vi "Autonomous Independent.vi"   [LabVIEW 2020]
doc: "This VI is called when autonomous begins, and will automatically be terminated when autonomous ends. You can carry out timed or sensor driven robot movement independently without needing to return to the caller."
uses:
  <vilib>/Rock Robotics/WPI/Solenoid/WPI_SolenoidValue.ctl
  <vilib>/Rock Robotics/WPI/Utilities/WPI_GetSetVariantRefNum.vi
  <vilib>/Rock Robotics/Network Tables/NT Read String.vi
  <vilib>/Rock Robotics/Network Tables/NT Write Numeric Array.vi
  Robot Global Data.vi
  <vilib>/Rock Robotics/Network Tables/NT Read Boolean.vi
  <vilib>/Rock Robotics/Network Tables/NT Read Number.vi
  Dawgma Programming Library/Utilities/armSetpoints.vi
  <vilib>/Rock Robotics/WPI/Solenoid/WPI_SolenoidSetEnum.vi
panel:
  # "Math for the\nfirst operation"
types:
  T1 = typedef "WPI_JoystickDevRef.ctl" = cluster{"Device":T2}
  T2 = typedef "WPI_JoystickDeviceEnum.ctl" = enum16{"USB 0", "USB 1", "USB 2", "USB 3", "USB 4", "USB 5"}
  T3 = typedef "WPI_SolenoidValue.ctl" = enum16{"Off", "On", "Forward", "Reverse"}
  T4 = typedef "Trajectory_Library.lvlib/SWERVE_DRIVE_ODOMETRY.ctl" = cluster{"POSE":T5, "GyroOffset":T7, "PreviousAngle":T7, "PrevModulePositions":T8[], "NumModules":i32}
  T5 = typedef "Trajectory_Library.lvlib/POSE2D.ctl" = cluster{"TRANSLATION":T6, "ROTATION":T7}
  T6 = typedef "Trajectory_Library.lvlib/TRANSLATION2D.ctl" = cluster{"X":dbl, "Y":dbl}
  T7 = typedef "Trajectory_Library.lvlib/ROTATION2D.ctl" = cluster{"VALUE":dbl, "COS":dbl, "SIN":dbl}
  T8 = typedef "Trajectory_Library.lvlib/SWERVE_DRIVE_MODULE_POSITION.ctl" = cluster{"Distance":dbl, "Angle":T7, "P":bool}
  T9 = typedef "WPI_SolenoidDevRef.ctl" = cluster{"DevStatus":errorcluster, "Pneumatics Control Module":u8, "Forward Solenoid Channel":T10, "Reverse Solenoid Channel":T10}
  T10 = typedef "WPI_SolenoidChannel.ctl" = enum8{"Solenoid 0", "Solenoid 1", "Solenoid 2", "Solenoid 3", "Solenoid 4", "Solenoid 5", "Solenoid 6", "Solenoid 7", "Solenoid 8", "Solenoid 9", "Solenoid 10", "Solenoid 11", "Solenoid 12", "Solenoid 13", "Solenoid 14", "Solenoid 15", "Invalid"}
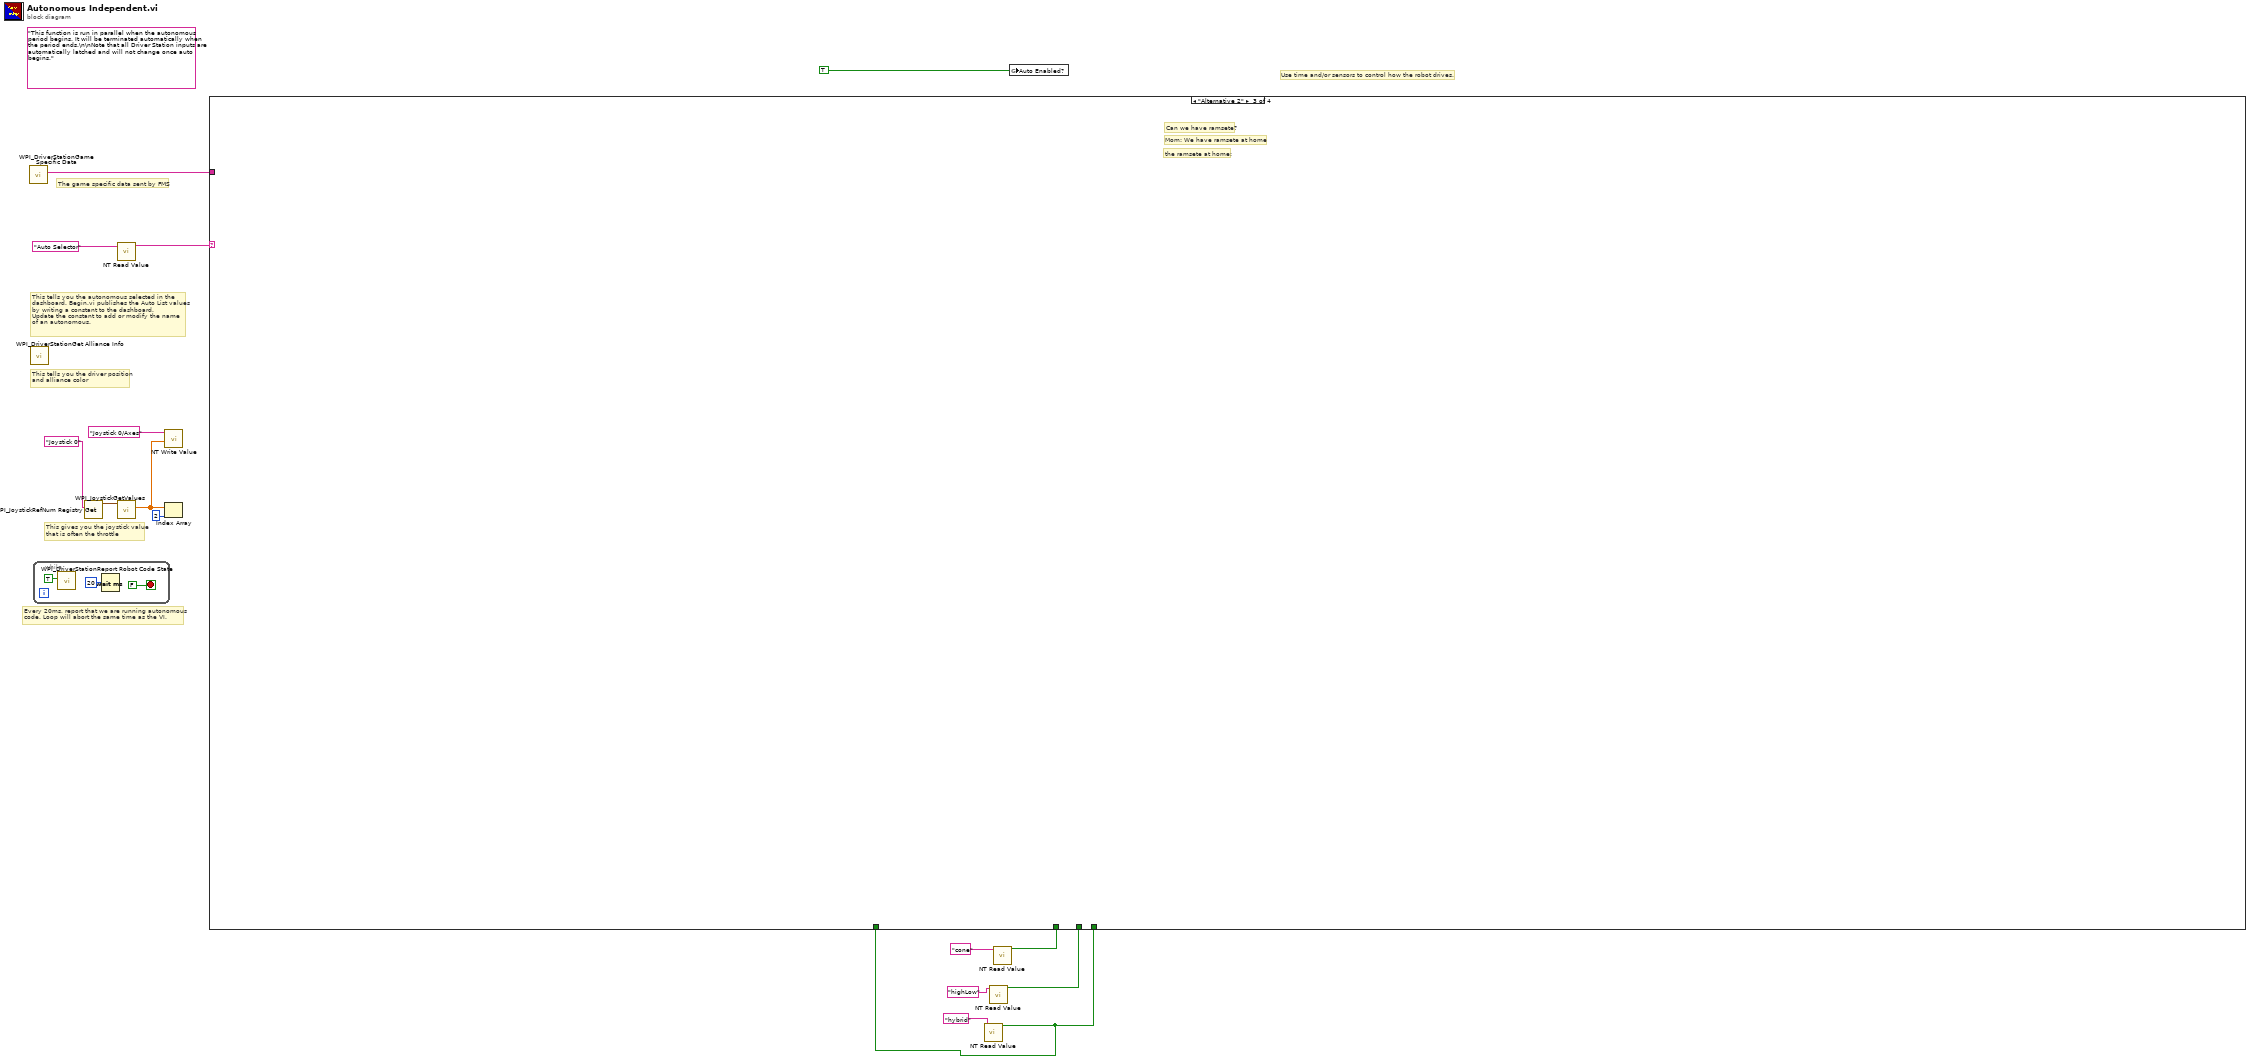
[diagram p0: block diagram]
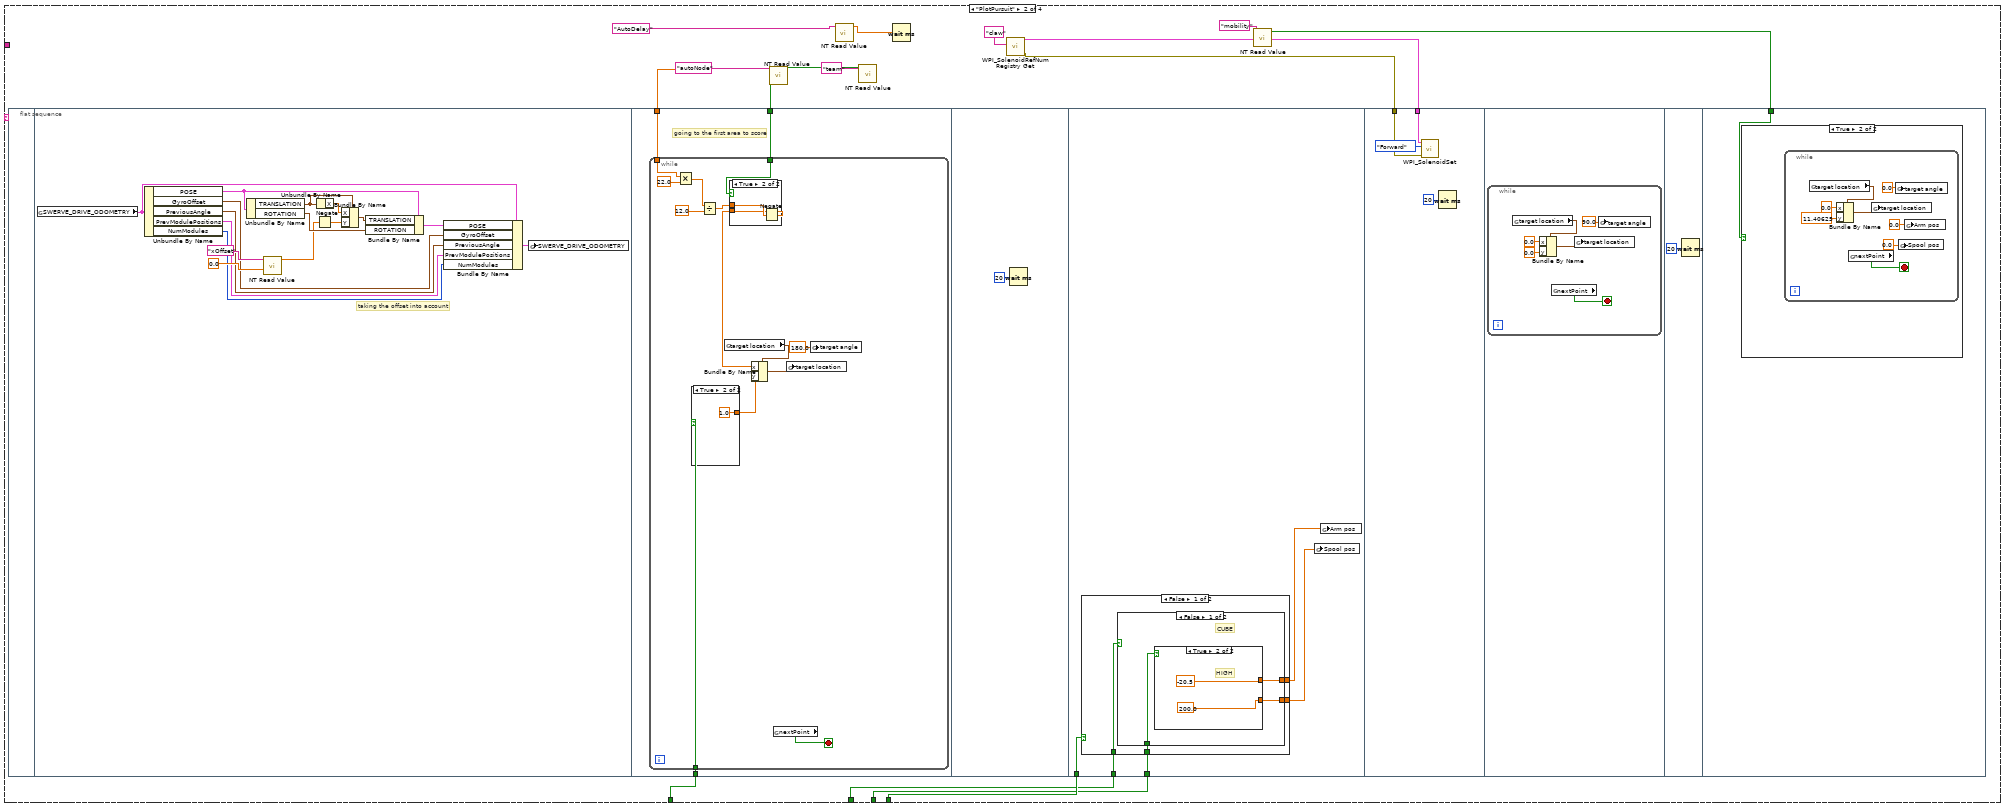
[diagram p3: hidden frame]
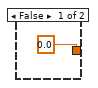
[diagram p4: hidden frame]
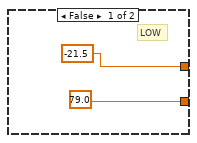
[diagram p6: hidden frame]
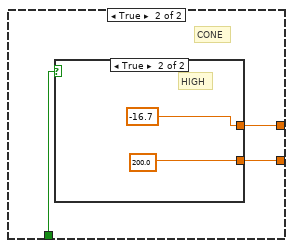
[diagram p7: hidden frame]
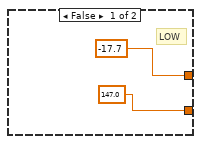
[diagram p8: hidden frame]
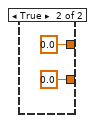
[diagram p9: hidden frame]
diagram:
  (unwired) "This function is run in parallel when the autonomous period begins. It will be terminated automatically when the period ends.\n\nNote that all Driver Station inputs are automatically latched and will not change once auto begins."
  # "The game specific data sent by FMS"
  # "This tells you the autonomous selected in the \ndashboard. Begin.vi publishes the Auto List values\nby writing a constant to the dashboard.\nUpdate the constant to add or modify the name\nof an autonomous."
  # "Every 20ms, report that we are running autonomous\ncode. Loop will abort the same time as the VI."
  # "This gives you the joystick value\nthat is often the throttle"
  # "Use time and/or sensors to control how the robot drives."
  # "This tells you the driver position\nand alliance color"
  n1 = call <vilib>:"WPI_DriverStationGame Specific Data.vi"() -> ("Game Specific Data"=w8:string)  [unwired: 11 in]
  n2 = call <vilib>:"WPI_DriverStationGet Alliance Info.vi"() -> ()  [unwired: 12 out]
  n3 = while {
    stop <- FALSE stop-if-true
    n4 = call <vilib>:"WPI_DriverStationReport Robot Code State.vi"("Autonomous"=TRUE) -> ()  [unwired: 10 in, 1 out]
    n5 = Wait (ms)(milliseconds to wait=u32 20) -> ()  [unwired: 1 out]
  }
  n6 = call <vilib>:"WPI_JoystickRefNum Registry Get.vi"("refnum name"="Joystick 0") -> ("JoystickDevRef"=w14:T1)  [unwired: 1 in, 9 out]
  n7 = call-poly <vilib>:"NT Read Value.vi"("name"="Auto Selector" ("Name")) -> ("value"=w11:string)  [unwired: 8 in, 2 out]
  n8 = call <vilib>:"WPI_JoystickGetValues.vi"("JoystickDevRef"=w14) -> ("Axes"=w10:dbl[])  [unwired: 6 in, 4 out]
  n9 = call-poly <vilib>:"NT Write Value.vi"("value"=w10, "name"="Joystick 0/Axes" ("Name")) -> ()  [unwired: 9 in, 1 out]
  n10 = Index Array(array=w10, index=2) -> ()  [unwired: 1 out]
  n11 = call-poly <vilib>:"NT Read Value.vi"("name"="hybrid") -> ("value"=w1:bool)  [unwired: 8 in, 2 out]
  n12 = call-poly <vilib>:"NT Read Value.vi"("name"="highLow") -> ("value"=w3:bool)  [unwired: 8 in, 2 out]
  n13 = call-poly <vilib>:"NT Read Value.vi"("name"="cone") -> ("value"=w5:bool)  [unwired: 8 in, 2 out]
  n14 = case shown="\"Alternative 2\"" w11 {
    tunnel: w8 -> [_ _ _ _]
    tunnel: w5 -> [_ w21 _ _]
    tunnel: w3 -> [_ w20 _ _]
    tunnel: w1 -> [_ w22 _ _]
    tunnel: w1 -> [_ w19 _ _]
    frame Default {
      # "You can put your main auto here, or you can right-click on the case and make any\nother frame be the default case."
      # "This is the frame that will execute if no selection is made, or if it is not recognized"
    }
    frame "PlotPursuit" {
      n15 = flat-sequence {
        tunnel: w27 -> [w52]
        tunnel: w25 -> [w51]
        tunnel: w19 -> [w50]
        tunnel: w22 -> [w74]
        tunnel: w21 -> [w73]
        tunnel: w20 -> [w72]
        tunnel: w30 -> [w99]
        tunnel: w29 -> [w98]
        tunnel: w23 -> [w108]
        frame #0 {
        }
        frame #1 {
          # "taking the offset into account"
          n16 = global read "Robot Global Data.vi" "SWERVE_DRIVE_ODOMETRY"() -> (w46:T4)
          n17 = Unbundle By Name(w46) -> ("POSE"=w41:T5, "GyroOffset"=w42:T7, "PreviousAngle"=w43:T7, "PrevModulePositions"=w44:T8[], "NumModules"=w45:i32)
          n18 = Unbundle By Name(w41) -> ("TRANSLATION"=w39:T6, "ROTATION"=w40:T7)
          n19 = call-poly <vilib>:"NT Read Value.vi"("default value"=0.0, "name"="xOffset") -> ("value"=w36:dbl)  [unwired: 7 in, 2 out]
          n20 = Negate(x=w36) -> (-x=w37:dbl)
          n21 = Unbundle By Name(w39) -> ("X"=w38:dbl)
          n22 = Bundle By Name(cluster=w39, "X"=w38, "Y"=w37) -> (w35:T6)
          n23 = Bundle By Name(cluster=w41, "TRANSLATION"=w35, "ROTATION"=w40) -> (w34:T5)
          n24 = Bundle By Name(cluster=w46, "POSE"=w34, "GyroOffset"=w42, "PreviousAngle"=w43, "PrevModulePositions"=w44, "NumModules"=w45) -> (w47:T4)
          n25 = global write "Robot Global Data.vi" "SWERVE_DRIVE_ODOMETRY"(w47) -> ()
        }
        frame #2 {
          # "going to the first area to score"
          n26 = while {
            tunnel: w52 -> [w58]
            tunnel: w51 -> [w55]
            tunnel: w50 -> [w54]
            stop <- w65 stop-if-true
            n27 = Multiply(x=w58, y=22.0) -> (x*y=w60:dbl)
            n28 = case shown="True" w54 {
              tunnel: [0.0 ("y") 1.0 ("y")] -> w53
              frame False {
              }
              frame True {
              }
            }
            n29 = Divide(x=w60, y=12.0) -> (x/y=w57:dbl)
            n30 = global read "Robot Global Data.vi" "target location"() -> (w62:cluster{"x":dbl, "y":dbl})
            n31 = case shown="True" w55 {
              tunnel: w57 -> [w68 w70]
              tunnel: [w68 w69] -> w56
              frame False {
              }
              frame True {
                n32 = Negate(x=w70) -> (-x=w69:dbl)
              }
            }
            n33 = Bundle By Name(cluster=w62, "x"=w56, "y"=w53) -> (w63:cluster{"x":dbl, "y":dbl})
            n34 = global read "Robot Global Data.vi" "nextPoint"() -> (w65:bool)
            n35 = global write "Robot Global Data.vi" "target location"(w63) -> ()
            n36 = global write "Robot Global Data.vi" "target angle"(180.0 ("target angle")) -> ()
          }
        }
        frame #3 {
          n37 = Wait (ms)(milliseconds to wait=u32 20) -> ()  [unwired: 1 out]
        }
        frame #4 {
          n38 = case shown="False" w74 {
            tunnel: [w80 0.0 ("Arm pos")] -> w76
            tunnel: [w79 0.0 ("Spool pos")] -> w75
            tunnel: w73 -> [w78 _]
            tunnel: w72 -> [w77 _]
            frame False {
              n39 = case shown="False" w78 {
                tunnel: [w83 w90] -> w80
                tunnel: [w82 w89] -> w79
                tunnel: w77 -> [w81 w88]
                frame False {
                  # "CUBE"
                  n40 = case shown="True" w81 {
                    tunnel: [-21.5 ("Arm pos") -20.5 ("Arm pos")] -> w83
                    tunnel: [79.0 ("Spool pos") 200.0 ("Spool pos")] -> w82
                    frame False {
                      # "LOW"
                    }
                    frame True {
                      # "HIGH"
                    }
                  }
                }
                frame True {
                  # "CONE"
                  n41 = case shown="True" w88 {
                    tunnel: [-17.7 ("Arm pos") -16.7 ("Arm pos")] -> w90
                    tunnel: [147.0 ("Spool pos") 200.0 ("Spool pos")] -> w89
                    frame False {
                      # "LOW"
                    }
                    frame True {
                      # "HIGH"
                    }
                  }
                }
              }
            }
            frame True {
            }
          }
          n42 = global write "armSetpoints.vi" "Spool pos"(w75) -> ()
          n43 = global write "armSetpoints.vi" "Arm pos"(w76) -> ()
        }
        frame #5 {
          n44 = call-poly <vilib>:"WPI_SolenoidSet.vi"("error in (no error)"=w98, "Value"=WPI_SolenoidValue."Forward", "SolenoidDevRef"=w99) -> ()  [unwired: 7 in, 2 out]
          n45 = Wait (ms)(milliseconds to wait=u32 20) -> ()  [unwired: 1 out]
        }
        frame #6 {
          n46 = while {
            stop <- w106 stop-if-true
            n47 = global read "Robot Global Data.vi" "target location"() -> (w103:cluster{"x":dbl, "y":dbl})
            n48 = Bundle By Name(cluster=w103, "x"=0.0, "y"=0.0) -> (w104:cluster{"x":dbl, "y":dbl})
            n49 = global read "Robot Global Data.vi" "nextPoint"() -> (w106:bool)
            n50 = global write "Robot Global Data.vi" "target location"(w104) -> ()
            n51 = global write "Robot Global Data.vi" "target angle"(90.0 ("target angle")) -> ()
          }
        }
        frame #7 {
          n52 = Wait (ms)(milliseconds to wait=u32 20) -> ()  [unwired: 1 out]
        }
        frame #8 {
          n53 = case shown="True" w108 {
            frame False {
            }
            frame True {
              n54 = while {
                stop <- w116 stop-if-true
                n55 = global read "Robot Global Data.vi" "target location"() -> (w113:cluster{"x":dbl, "y":dbl})
                n56 = Bundle By Name(cluster=w113, "x"=0.0, "y"=11.40625) -> (w114:cluster{"x":dbl, "y":dbl})
                n57 = global read "Robot Global Data.vi" "nextPoint"() -> (w116:bool)
                n58 = global write "Robot Global Data.vi" "target location"(w114) -> ()
                n59 = global write "Robot Global Data.vi" "target angle"(0.0 ("target angle")) -> ()
                n60 = global write "armSetpoints.vi" "Spool pos"(0.0 ("Spool pos")) -> ()
                n61 = global write "armSetpoints.vi" "Arm pos"(0.0 ("Arm pos")) -> ()
              }
            }
          }
        }
      }
      n62 = call-poly <vilib>:"NT Read Value.vi"("name"="autoNode") -> ("value"=w27:dbl)  [unwired: 8 in, 2 out]
      n63 = call-poly <vilib>:"NT Read Value.vi"("name"="AutoDelay") -> ("value"=w32:dbl)  [unwired: 8 in, 2 out]
      n64 = call-poly <vilib>:"NT Read Value.vi"("name"="team") -> ("value"=w25:bool)  [unwired: 8 in, 2 out]
      n65 = Wait (ms)(milliseconds to wait=w32) -> ()  [unwired: 1 out]
      n66 = call <vilib>:"WPI_SolenoidRefNum Registry Get.vi"("refnum name"="claw") -> ("error out"=w29:errorcluster, "SolenoidDevRef"=w30:T9)  [unwired: 9 in]
      n67 = call-poly <vilib>:"NT Read Value.vi"("name"="mobility") -> ("value"=w23:bool)  [unwired: 8 in, 2 out]
    }
    frame "Alternative 2" {
      # "the ramsete at home:"
      # "Mom: We have ramsete at home"
      # "Can we have ramsete?"
    }
    frame "Your Turn" {
    }
  }
  n68 = global write "Robot Global Data.vi" "Auto Enabled?"(TRUE ("Auto Enabled?")) -> ()
